vi "CSV Reader.vi"(8 "error in (no error)":errorcluster, 11 "CSV Reader Inputs":T2={"Frequency Type"=enum."Frequency", "Measurement Type"=enum."Power", "Digital Channel Selector"=enum."2", "OGE Type"=enum."OGnE", "CSV File Input"=path ""}) -> (0 "error out":errorcluster, 3 "Terminals":T1[](array[typedef]))   [LabVIEW 2017]
uses:
  CSV Reader Inputs.ctl
  Frequency_Type.ctl
  Measurement_Type.ctl
  Digital Channel Selector.ctl
  Terminal Data.ctl
  <vilib>/Utility/file.llb/Read Delimited Spreadsheet (string).vi
panel:
  in  "stop":bool
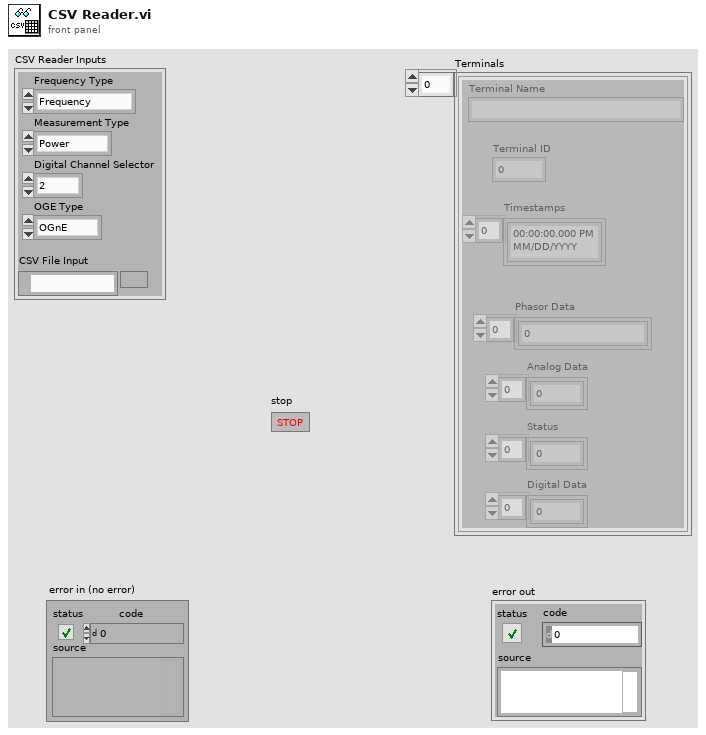
[diagram p1: front panel]
types:
  T1 = typedef "Terminal Data.ctl" = cluster{"Terminal Name":string, "Terminal ID":dbl, "Timestamps":timestamp[], "Phasor Data":cdb[], "Analog Data":dbl[], "Status":dbl[], "Digital Data":dbl[]}
  T2 = typedef "CSV Reader Inputs.ctl" = cluster{"Frequency Type":T3, "Measurement Type":T4, "Digital Channel Selector":T5, "OGE Type":enum16{"WAN OGE", "OGnE"}, "CSV File Input":path}
  T3 = typedef "Frequency_Type.ctl" = enum16{"Frequency", "df/dt"}
  T4 = typedef "Measurement_Type.ctl" = enum16{"Voltage", "Current", "Power"}
  T5 = typedef "Digital Channel Selector.ctl" = enum16{"1", "2", "3"}
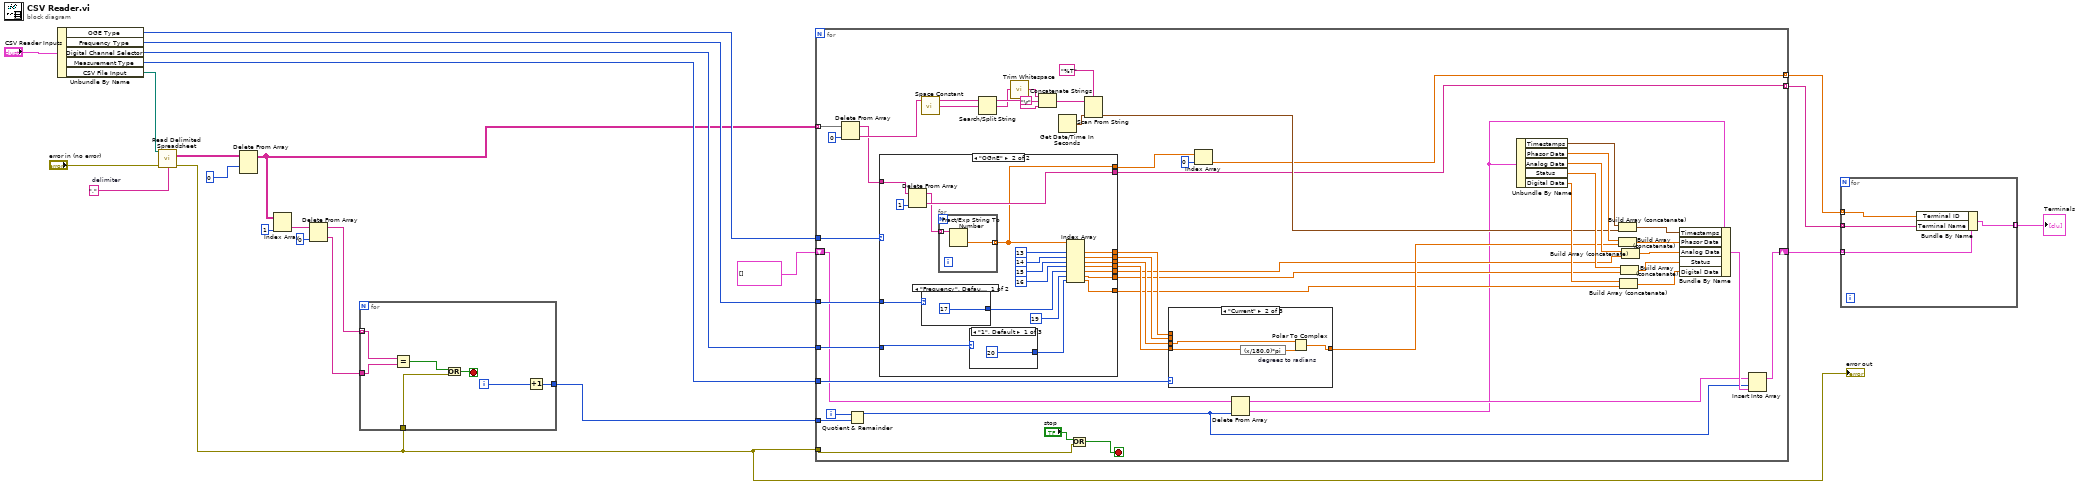
[diagram p0: block diagram]
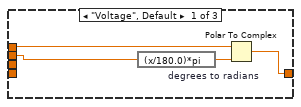
[diagram p2: hidden frame]
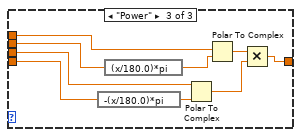
[diagram p3: hidden frame]
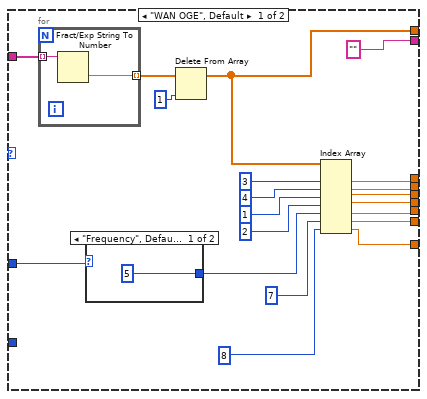
[diagram p4: hidden frame]
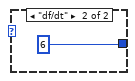
[diagram p5: hidden frame]
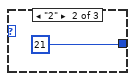
[diagram p6: hidden frame]
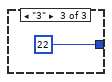
[diagram p7: hidden frame]
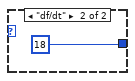
[diagram p8: hidden frame]
diagram:
  w23 = ","  # delimiter
  n1 = Unbundle By Name("CSV Reader Inputs") -> ("OGE Type"=w19:enum16{"WAN OGE", "OGnE"}, "Frequency Type"=w18:T3, "Digital Channel Selector"=w17:T5, "Measurement Type"=w16:T4, "CSV File Input"=w1:path)
  n2 = call-poly <vilib>:"Read Delimited Spreadsheet.vi"("file path (dialog if empty)"=w1, "error in (no error)"="error in (no error)", "delimiter (\\t)"=w23) -> ("all rows"=w22:string[][], "error out"=w7:errorcluster)  [unwired: 7 in, 4 out]
  "error out" <- w7
  n3 = Delete From Array(array=w22, index (row)=0) -> (array with subset deleted=w14:string[][])  [unwired: 2 in, 1 out]
  n4 = Index Array(array=w14, index (col)=1 ("disabled index (col)")) -> (element=w12:string[])  [unwired: 1 in]
  n5 = Delete From Array(array=w12, index=0) -> (deleted portion=w9:string, array with subset deleted=w10:string[])  [unwired: 1 in]
  n6 = for {
    tunnel: w10 -> [w28] mode=indexing
    tunnel: w9 -> [w27]
    tunnel: [w29] -> w8
    tunnel: w7 -> [w26]
    i -> [w30]
    stop <- w24 stop-if-true
    n7 = Equal?(x=w28, y=w27) -> (x = y?=w25:bool)
    n8 = Or(x=w25, y=w26) -> (x .or. y?=w24:bool)
    n9 = Increment(x=w30) -> (x+1=w29:i32)
  }
  n10 = for {
    tunnel: w14 -> [w72] mode=indexing
    tunnel: w19 -> [w68]
    tunnel: w16 -> [w65]
    tunnel: w18 -> [w60]
    tunnel: w17 -> [w59]
    tunnel: w7 -> [w36]
    shift-right: [w42] -> w5
    shift-left: T1[] [] ("Terminals 2") -> [w40]
    tunnel: w8 -> [w38]
    tunnel: [w32] -> w3 mode=indexing
    tunnel: [w31] -> w4 mode=indexing
    i -> [w44]
    stop <- w35 stop-if-true
    n11 = Delete From Array(array=w72, index=0) -> (deleted portion=w70:string, array with subset deleted=w69:string[])  [unwired: 1 in]
    n12 = Quotient & Remainder(x=w44, y=w38) -> (x-y*floor(x/y)=w39:i32)  [unwired: 1 out]
    n13 = case shown="\"OGnE\"" w68 {
      tunnel: w69 -> [w117 w141]
      tunnel: ["" ("String") w140] -> w31
      tunnel: [w98 w138] -> w67
      tunnel: [w108 w133] -> w64
      tunnel: [w107 w132] -> w63
      tunnel: [w106 w131] -> w62
      tunnel: [w105 w130] -> w61
      tunnel: w60 -> [w109 w129]
      tunnel: [w104 w127] -> w50
      tunnel: w59 -> [_ w125]
      tunnel: [w103 w123] -> w48
      tunnel: [w102 w122] -> w46
      frame "WAN OGE", Default {
        n14 = for {
          tunnel: [w120] -> w100 mode=indexing
          tunnel: w117 -> [w121] mode=indexing
          n15 = Fract/Exp String To Number(string=w121) -> (number=w120:dbl)  [unwired: 3 in, 1 out]
        }
        n16 = case shown="\"Frequency\", Default" w109 {
          tunnel: [5 ("index") 6 ("index")] -> w111
          frame "Frequency", Default {
          }
          frame "df/dt" {
          }
        }
        n17 = Delete From Array(array=w100, index=1) -> (array with subset deleted=w98:dbl[])  [unwired: 1 in, 1 out]
        n18 = Index Array(array=w98, index #1=3 ("index"), index #2=4 ("index"), index #3=1 ("index"), index #4=2 ("index"), index #5=w111, index #6=7 ("index"), index #7=8 ("index")) -> (element #1=w108:dbl, element #2=w107:dbl, element #3=w106:dbl, element #4=w105:dbl, element #5=w104:dbl, element #6=w103:dbl, element #7=w102:dbl)
      }
      frame "OGnE" {
        n19 = Delete From Array(array=w141, index=1) -> (deleted portion=w140:string, array with subset deleted=w139:string[])  [unwired: 1 in]
        n20 = case shown="\"Frequency\", Default" w129 {
          tunnel: [17 ("index") 18 ("index")] -> w128
          frame "Frequency", Default {
          }
          frame "df/dt" {
          }
        }
        n21 = for {
          tunnel: [w148] -> w138 mode=indexing
          tunnel: w139 -> [w149] mode=indexing
          n22 = Fract/Exp String To Number(string=w149) -> (number=w148:dbl)  [unwired: 3 in, 1 out]
        }
        n23 = case shown="\"1\", Default" w125 {
          tunnel: [20 ("index") 21 ("index") 22 ("index")] -> w124
          frame "1", Default {
          }
          frame "2" {
          }
          frame "3" {
          }
        }
        n24 = Index Array(array=w138, index #1=13 ("index"), index #2=14 ("index"), index #3=15 ("index"), index #4=16 ("index"), index #5=w128, index #6=19 ("index"), index #7=w124) -> (element #1=w133:dbl, element #2=w132:dbl, element #3=w131:dbl, element #4=w130:dbl, element #5=w127:dbl, element #6=w123:dbl, element #7=w122:dbl)
      }
    }
    n25 = call <vilib>:"Space Constant.vi"() -> ("String"=w76:string)
    n26 = Search/Split String(string=w70, search string/char (-)=w76) -> (substring before match=w78:string, match + rest of string=w77:string)  [unwired: 1 in, 1 out]
    n27 = call <vilib>:"Trim Whitespace.vi"("string"=w77) -> ("trimmed string"=w79:string)  [unwired: 1 in]
    n28 = Concatenate Strings(w79, "\r", w78) -> (w80:string)
    n29 = Get Date/Time In Seconds() -> (seconds since 1Jan1904=w75:timestamp)
    n30 = Or(x="stop", y=w36) -> (x .or. y?=w35:bool)
    n31 = Scan From String(format string="%T", input string=w80, default 1=w75) -> (output 1=w53:timestamp)  [unwired: 2 in, 3 out]
    n32 = case shown="\"Current\"" w65 {
      tunnel: w64 -> [w83 _ w93]
      tunnel: w63 -> [w82 _ w92]
      tunnel: w62 -> [_ w86 w91]
      tunnel: w61 -> [_ w85 w90]
      tunnel: [w81 w87 w89] -> w52
      frame "Voltage", Default {
        n33 = expression code="(x/180.0)*pi" "degrees to radians"(w82) -> (w84:dbl)
        n34 = Polar To Complex(1:w84, 2:w83) -> (0:w81:cdb)
      }
      frame "Current" {
        n35 = expression code="(x/180.0)*pi" "degrees to radians"(w85) -> (w88:dbl)
        n36 = Polar To Complex(1:w88, 2:w86) -> (0:w87:cdb)
      }
      frame "Power" {
        n37 = expression code="-(x/180.0)*pi" ("degrees to radians")(w90) -> (w97:dbl)
        n38 = expression code="(x/180.0)*pi" ("degrees to radians")(w92) -> (w95:dbl)
        n39 = Polar To Complex(1:w97, 2:w91) -> (0:w96:cdb)
        n40 = Polar To Complex(1:w95, 2:w93) -> (0:w94:cdb)
        n41 = Multiply(x=w94, y=w96) -> (x*y=w89:cdb)
      }
    }
    n42 = Index Array "Index Array"(array=w67, index=0) -> (element=w32:dbl)
    n43 = Delete From Array(array=w40, index=w39) -> (deleted portion=w33:T1, array with subset deleted=w37:T1[])  [unwired: 1 in]
    n44 = Unbundle By Name(w33) -> ("Timestamps"=w58:timestamp[], "Phasor Data"=w57:cdb[], "Analog Data"=w56:dbl[], "Status"=w55:dbl[], "Digital Data"=w54:dbl[])
    n45 = Build Array (concatenate)(w58, w53) -> (w43:timestamp[])
    n46 = Build Array (concatenate)(w57, w52) -> (w51:cdb[])
    n47 = Build Array (concatenate)(w54, w46) -> (w45:dbl[])
    n48 = Build Array (concatenate)(w55, w48) -> (w47:dbl[])
    n49 = Build Array (concatenate)(w56, w50) -> (w49:dbl[])
    n50 = Bundle By Name(cluster=w33, "Timestamps"=w43, "Phasor Data"=w51, "Analog Data"=w49, "Status"=w47, "Digital Data"=w45) -> (w41:T1)
    n51 = Insert Into Array(array=w37, index=w39, new element=w41) -> (w42:T1[])
  }
  n52 = for {
    tunnel: w5 -> [w151] mode=indexing
    tunnel: w4 -> [w152] mode=indexing
    tunnel: w3 -> [w153] mode=indexing
    tunnel: [w150] -> w2 mode=indexing
    n53 = Bundle By Name(cluster=w151, "Terminal ID"=w153, "Terminal Name"=w152) -> (w150:T1)
  }
  "Terminals" <- w2
